vi "Tbl_Add (SubVI).vi"(10 "meas":string[](array[string]), 11 "Table in":refnum<vi>) -> (3 "element":i32)   [LabVIEW 2017]
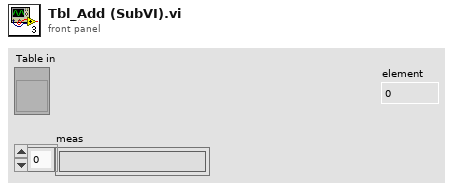
[diagram p1: front panel]
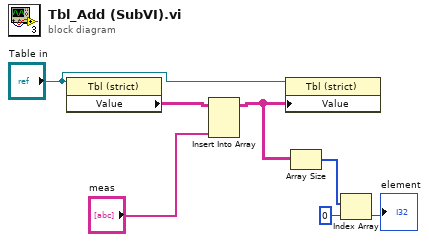
[diagram p0: block diagram]
diagram:
  n1 = property class="Tbl (strict)"(reference="Table in") -> ("Value"=w7:string[][])  [unwired: 1 in, 2 out]
  n2 = Insert Into Array(array=w7, new element="meas") -> (w4:string[][])  [unwired: 2 in]
  n3 = property class="Tbl (strict)"(reference="Table in", "Value"=w4) -> ()  [unwired: 1 in, 2 out]
  n4 = Array Size(array=w4) -> (size(s)=w3:i32[])
  n5 = Index Array(array=w3, index=0) -> (element=→"element":i32)
